vi "Progress bar.vi"(7 "Please wait...":u8(slide) max=1 scale=0.0..100.0) -> ()   [LabVIEW 2017]
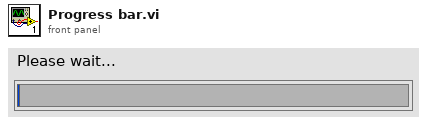
[diagram p1: front panel]
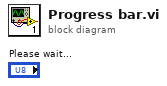
[diagram p0: block diagram]
diagram:
